vi "Set Safe State.vi"(8 "error in":errorcluster, 9 "timeout (-1)":i32=-1, 11 "Engine Runtime Interface in":refnum<class "Engine Runtime Interface.lvclass">) -> (0 "error out":errorcluster, 3 "Engine Runtime Interface out":refnum<class "Engine Runtime Interface.lvclass">)   [LabVIEW 2013, in "Engine Runtime Interface.lvclass"]
doc: "This function transitions an engine from the running state to its configured safe-state."
uses:
  Engine Runtime Interface.lvclass
  <vilib>/NI/Configuration Framework/NISE_CEF_TreeControl.lvlib
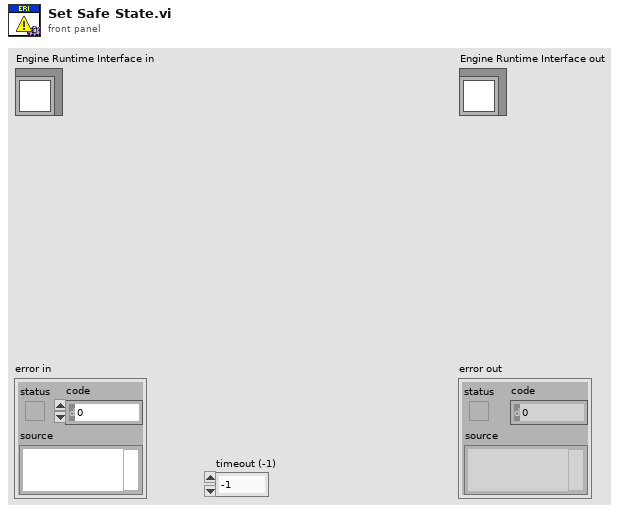
[diagram p1: front panel]
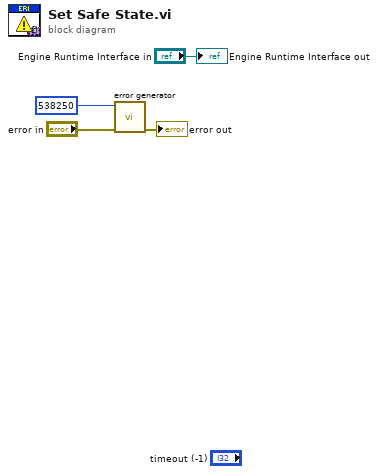
[diagram p0: block diagram]
diagram:
  n1 = call <vilib>:"error generator.vi"("error in"="error in", "error code (0)"=538250) -> ("error out"=→"error out":errorcluster)  [unwired: 7 in]
  "Engine Runtime Interface out" <- "Engine Runtime Interface in"
